vi "DVR_Update.vi"(10 "Numeric":dbl, 11 "DataValRefNum in":refnum<vi>) -> ()   [LabVIEW 2025]
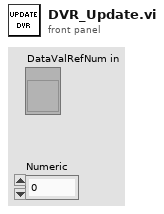
[diagram p1: front panel]
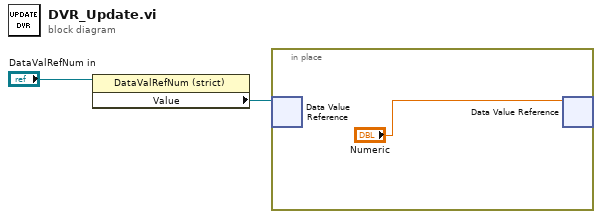
[diagram p0: block diagram]
diagram:
  n1 = property class="DataValRefNum (strict)"(reference="DataValRefNum in") -> ("Value"=w2:refnum<data-value>)  [unwired: 1 in, 2 out]
  n2 = in-place {
    n3 = in-place-dvr #1(w2) -> ()  [unwired: 2 out]
    n4 = in-place-dvr #1("Numeric") -> ()  [unwired: 2 out]
  }
